vi "DAQ-Scope Stitching API.vi"(8 "Error In":errorcluster, 9 "Scope Filename":string, 10 "DAQ Filename":string, 11 "File IO":T1={"Output Folder"=path "C:/Users/Abigail/Documents/Imperial Optical software/Optical Software Code Simplified/Output", "Error file"=path "Error Log.txt", "Config file"=path "Config.ini", "File prefix"="", "Waveform read"={"t0"=timestamp(0 s since 1904-01-01), "dt"=1.0, "Y"=[]}}) -> (0 "Error Out":errorcluster)   [LabVIEW 2017, in "Processing.lvlib"]
uses:
  Processing.lvlib
  File IO/Controls/Params.ctl
  Controls/Command Data [cluster].ctl
  Controls/Commands [enum].ctl
  Events/Events.lvlib
  File IO/File IO.lvlib
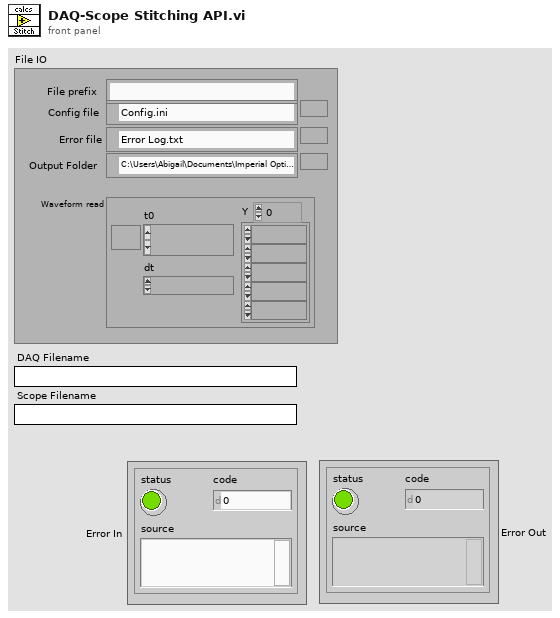
[diagram p1: front panel]
types:
  T1 = typedef "File IO.lvlib/Params.ctl" = cluster{"Output Folder":path, "Error file":path, "Config file":path, "File prefix":string, "Waveform read":waveform(dbl)}
  T2 = cluster{"File IO":T1, "Filename (A)":string, "Filename (B)":string}
  T3 = typedef "Processing.lvlib/Command Data [cluster].ctl" = cluster{"Command":T4, "Data":variant}
  T4 = typedef "Processing.lvlib/Commands [enum].ctl" = enum16{"Start", "Stop", "Process waveform", "Scope A-B processing", "DAQ A-B processing", "DAQ-Scope Stitching", "Update Test Info"}
  T5 = typedef "Events.lvlib/Refs [cluster].ctl" = cluster{"Exit":refnum<user-event>, "Controller":refnum<user-event>, "System Error":refnum<user-event>, "UI":refnum<user-event>, "Example Module":refnum<user-event>, "Shutter":refnum<user-event>, "Monochromator":refnum<user-event>, "DAQ":refnum<user-event>, "Scope":refnum<user-event>, "Processing":refnum<user-event>, "File IO":refnum<user-event>, "Colour wheel":refnum<user-event>}
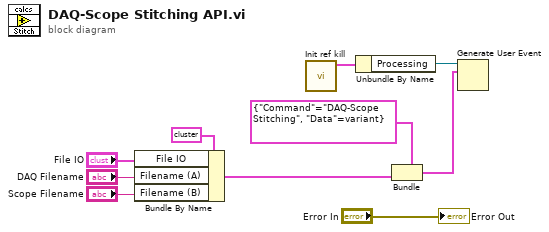
[diagram p0: block diagram]
diagram:
  n1 = Bundle By Name(cluster=T2 {"File IO"={"Output Folder"=path "", "Error file"=path "", "Config file"=path "", "File prefix"="", "Waveform read"={"t0"=timestamp(0 s since 1904-01-01), "dt"=1.0, "Y"=[]}}, "Filename (A)"="", "Filename (B)"=""}, "File IO"="File IO", "Filename (A)"="DAQ Filename", "Filename (B)"="Scope Filename") -> (w4:T2)
  n2 = call "Init ref kill.vi"() -> ("Messages"=w10:T5)  [unwired: 10 in, 1 out]
  n3 = Unbundle By Name(w10) -> ("Processing"=w9:refnum<user-event>)
  n4 = Bundle(cluster=T3 {"Command"=enum."DAQ-Scope Stitching", "Data"=variant} ("event data"), "Data"=w4) -> (w6:T3)  [unwired: 1 in]
  n5 = Generate User Event(user event=w9, event data cluster=w6) -> ()  [unwired: 2 in, 2 out]
  "Error Out" <- "Error In"
